vi "PH_Names.get Instance Name out of SM State Service.vi"(0 "Service Name SM State":string) -> (1 "Instance Name found":bool, 2 "Instance":string)   [LabVIEW 2014, in "PH_Common.lvlib"]
uses:
  PH_Common.lvlib
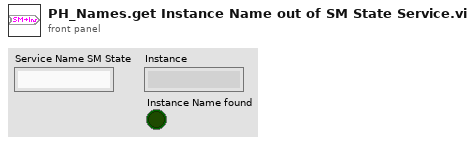
[diagram p1: front panel]
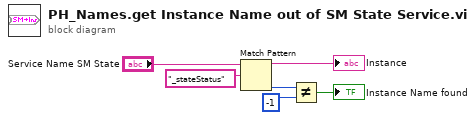
[diagram p0: block diagram]
diagram:
  n1 = Match Pattern(string="Service Name SM State", regular expression="_stateStatus") -> (before substring=→"Instance":string, offset past match=w3:i32)  [unwired: 1 in, 2 out]
  n2 = Not Equal?(x=w3, y=-1) -> (x != y?=→"Instance Name found":bool)
